vi "Summarize Desription.vi"(11 "Description in":string) -> (3 "Summary out":string)   [LabVIEW 2020]
doc: "This method summarizes the description by taking only the first sentance or first line of text from the description."
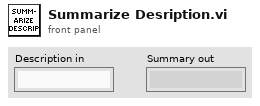
[diagram p1: front panel]
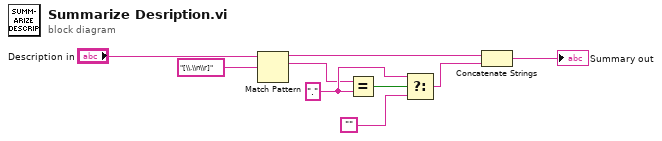
[diagram p0: block diagram]
diagram:
  w7 = "."
  n1 = Match Pattern(string="Description in", regular expression="[\\.\\n\\r]") -> (before substring=w2:string, match substring=w5:string)  [unwired: 1 in, 2 out]
  n2 = Equal?(x=w5, y=w7) -> (x = y?=w6:bool)
  n3 = Select(t=w7, s=w6, f="") -> (s? t:f=w8:string)
  n4 = Concatenate Strings(w2, w8) -> (→"Summary out":string)
